vi "Voltages_2_I16.vi"(0 "Voltages":dbl[][](array[numeric])) -> (1 "Group Channel Settings":T1(array[cluster]), 2 "I16 data":i16[][](array[numeric]))   [LabVIEW 2013]
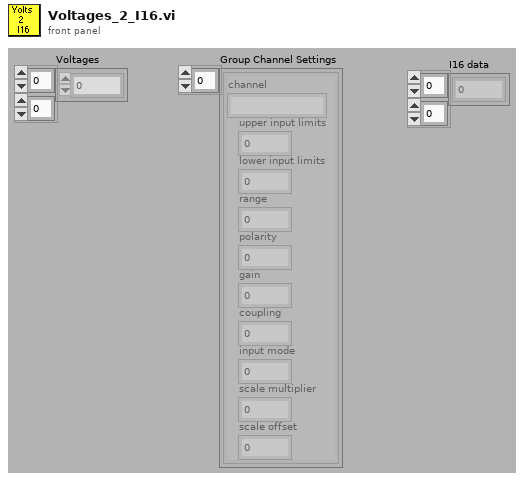
[diagram p1: front panel]
types:
  T1 = cluster{"channel":string, "upper input limits":sgl, "lower input limits":sgl, "range":sgl, "polarity":u16, "gain":sgl, "coupling":u16, "input mode":u16, "scale multiplier":dbl, "scale offset":dbl}[]
  T2 = cluster{"channel":string, "upper input limits":sgl, "lower input limits":sgl, "range":sgl, "polarity":u16, "gain":sgl, "coupling":u16, "input mode":u16, "scale multiplier":dbl, "scale offset":dbl}
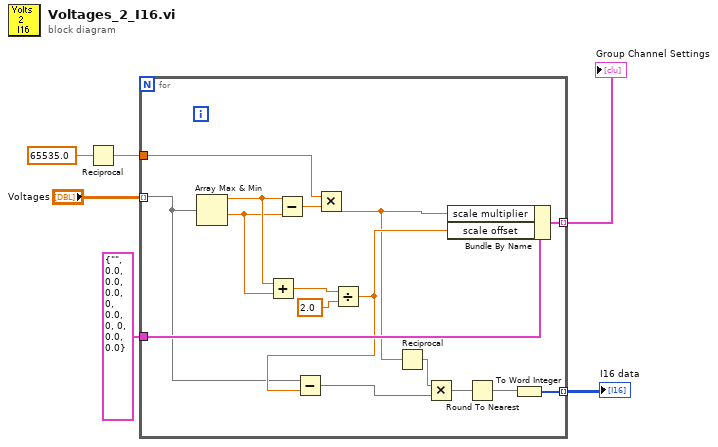
[diagram p0: block diagram]
diagram:
  n1 = Reciprocal(x=65535.0 ("y")) -> (1/x=w1:dbl)
  n2 = for {
    tunnel: T2 {"channel"="", "upper input limits"=0.0, "lower input limits"=0.0, "range"=0.0, "polarity"=0, "gain"=0.0, "coupling"=0, "input mode"=0, "scale multiplier"=0.0, "scale offset"=0.0} -> [w22]
    tunnel: [w21] -> w5 mode=indexing
    tunnel: [w16] -> w4 mode=indexing
    tunnel: "Voltages" -> [w14] mode=indexing
    tunnel: w1 -> [w11]
    n3 = Array Max & Min(array=w14) -> (max value=w20:dbl, min value=w19:dbl)  [unwired: 2 out]
    n4 = Add(x=w20, y=w19) -> (x+y=w18:dbl)
    n5 = Subtract(x=w20, y=w19) -> (x-y=w12:dbl)
    n6 = Multiply(x=w11, y=w12) -> (x*y=w10:dbl)
    n7 = Divide(x=w18, y=2.0) -> (x/y=w15:dbl)
    n8 = Subtract(x=w14, y=w15) -> (x-y=w8:dbl[])
    n9 = Reciprocal(x=w10) -> (1/x=w9:dbl)
    n10 = Multiply(x=w9, y=w8) -> (x*y=w7:dbl[])
    n11 = Bundle By Name(cluster=w22, "scale multiplier"=w10, "scale offset"=w15) -> (w21:T2)
    n12 = Round To Nearest(number=w7) -> (nearest integer value=w13:dbl[])
    n13 = To Word Integer(number=w13) -> (16bit integer=w16:i16[])
  }
  "Group Channel Settings" <- w5
  "I16 data" <- w4
